vi "IrCheckJumboFrame.vi"(8 "error in (no error)":errorcluster) -> (0 "error out":errorcluster, 2 "reboot required":bool)   [LabVIEW 2017]
uses:
  <vilib>/Utility/config.llb/NI_LVConfig.lvlib
  <vilib>/Utility/config.llb/Read Key (String).vi
  <vilib>/Utility/config.llb/Write Key (String).vi
panel:
  in  "Path":path
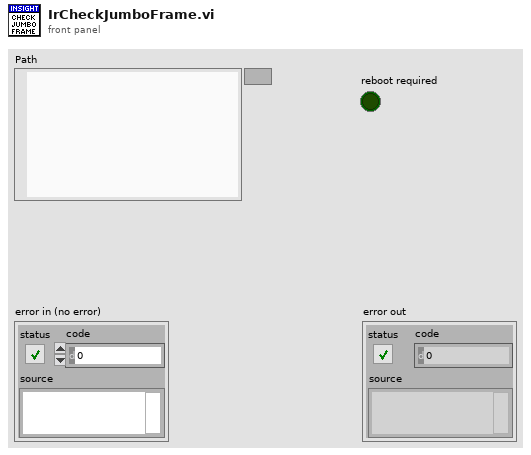
[diagram p1: front panel]
types:
  T1 = typedef "NI_LVConfig.lvlib/Config Data RefNum.ctl" = refnum<k1>
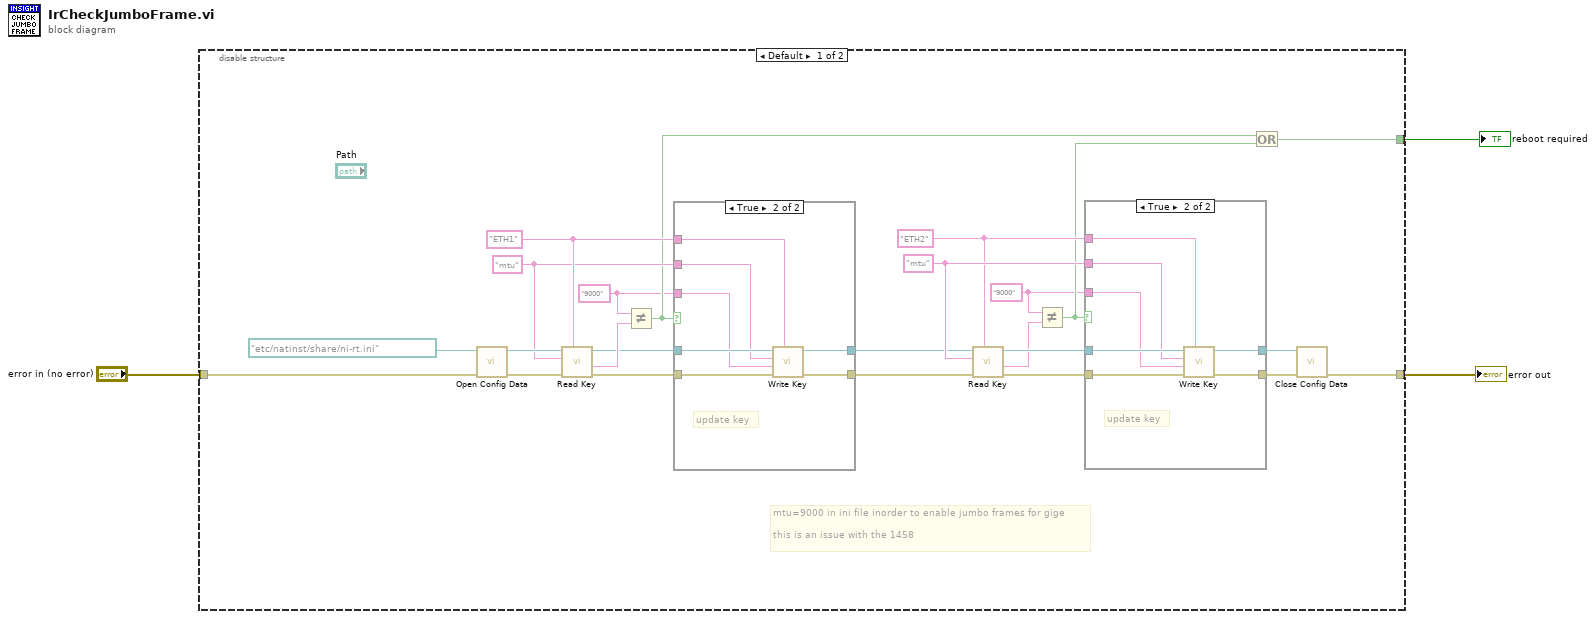
[diagram p0: block diagram]
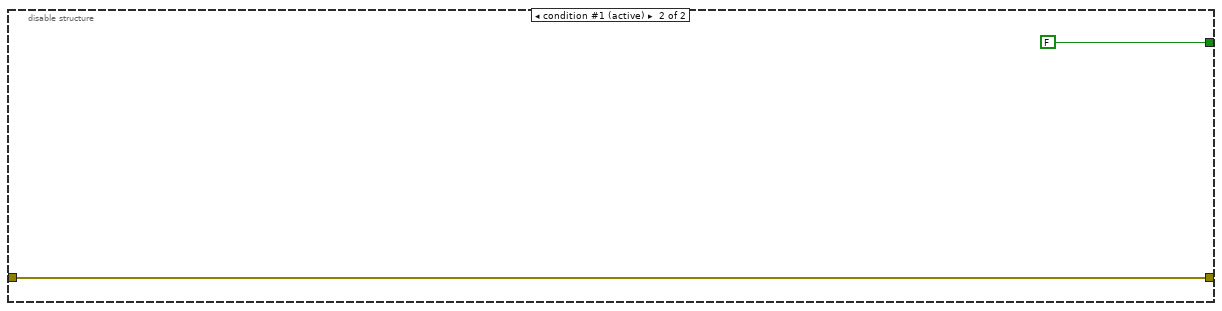
[diagram p4: hidden frame]
diagram:
  n1 = disable-structure shown="Default" {
    disable-tunnel: "error in (no error)" -> [w20 w47]
    disable-tunnel: [w10 w47] -> w2
    disable-tunnel: [w7 FALSE ("reboot required")] -> w1
    frame condition #0 {
      w5 = "9000" ("key")
      w6 = "9000" ("key")
      w19 = "mtu" ("key")
      w18 = "ETH2" ("section")
      w21 = "mtu" ("key")
      w22 = "ETH1" ("section")
      # "mtu=9000 in ini file inorder to enable jumbo frames for gige\n\nthis is an issue with the 1458"
      n2 = call <vilib>:"Open Config Data.vi"("error in (no error)"=w20, "configuration file path"=path "/etc/natinst/share/ni-rt.ini" ("Path")) -> ("error out"=w26:errorcluster, "refnum"=w27:T1)  [unwired: 7 in, 1 out]
      n3 = call-poly <vilib>:"Read Key.vi"("section"=w22, "error in (no error)"=w26, "key"=w21, "refnum"=w27) -> ("error out"=w24:errorcluster, "value"=w25:string, "refnum out"=w23:T1)  [unwired: 4 in, 1 out]
      n4 = Not Equal?(x=w6, y=w25) -> (x != y?=w8:bool)
      n5 = case shown="True" w8 {
        tunnel: w24 -> [w37 w44]
        tunnel: w23 -> [w38 w45]
        tunnel: [w38 w43] -> w14
        tunnel: [w37 w42] -> w13
        tunnel: w22 -> [_ w41]
        tunnel: w21 -> [_ w40]
        tunnel: w6 -> [_ w39]
        frame False {
        }
        frame True {
          # "update key"
          n6 = call-poly <vilib>:"Write Key.vi"("section"=w41, "error in (no error)"=w44, "value"=w39, "key"=w40, "refnum"=w45) -> ("error out"=w42:errorcluster, "refnum out"=w43:T1)  [unwired: 4 in, 1 out]
        }
      }
      n7 = call-poly <vilib>:"Read Key.vi"("section"=w18, "error in (no error)"=w13, "key"=w19, "refnum"=w14) -> ("error out"=w16:errorcluster, "value"=w15:string, "refnum out"=w17:T1)  [unwired: 4 in, 1 out]
      n8 = Not Equal?(x=w5, y=w15) -> (x != y?=w9:bool)
      n9 = case shown="True" w9 {
        tunnel: w16 -> [w28 w35]
        tunnel: w17 -> [w29 w36]
        tunnel: [w29 w34] -> w11
        tunnel: [w28 w33] -> w12
        tunnel: w18 -> [_ w32]
        tunnel: w19 -> [_ w31]
        tunnel: w5 -> [_ w30]
        frame False {
        }
        frame True {
          # "update key"
          n10 = call-poly <vilib>:"Write Key.vi"("section"=w32, "error in (no error)"=w35, "value"=w30, "key"=w31, "refnum"=w36) -> ("error out"=w33:errorcluster, "refnum out"=w34:T1)  [unwired: 4 in, 1 out]
        }
      }
      n11 = Or(x=w8, y=w9) -> (x .or. y?=w7:bool)
      n12 = call <vilib>:"Close Config Data.vi"("error in (no error)"=w12, "refnum"=w11) -> ("error out"=w10:errorcluster)  [unwired: 8 in, 1 out]
    }
    frame condition #1 (active) {
    }
  }
  "error out" <- w2
  "reboot required" <- w1
